vi "Hardware-RegisterControlsCalPoints.vi"(0 "User LED 1":T4, 1 "User LED 2":T4, 5 "Key [V]":sgl) -> (10 "System Settings":T5={"MPRD"=FALSE, "IO Lock MPRD Disable"=FALSE, "User LED 1"=enum."Off", "User LED 2"=enum."Off", "DI HS Fault Filter Time [s]"=1e-06, "Clamp Fault Filter Time [s]"=1e-06, "HH Shoot Through Time [s]"=1e-06, "HH ISeq Dur PS"=8, "HH Open Threshold [A]"=0.1} {"HH Open Threshold [A]" min=0 max=8 format="%#_3p"; "HH ISeq Dur PS" items=["3.3ms @ 20MHz"=0, "6.5ms @ 10MHz"=4, "13ms @ 5MHz"=6, "26ms @ 2.5MHz"=7]; "HH Shoot Through Time [s]" min=0 max=0.003277 format="%#_3p"; "Clamp Fault Filter Time [s]" min=0 max=0.003277 format="%#_3p"; "DI HS Fault Filter Time [s]" min=0 max=0.003277 format="%#_3p"}, 14 "A Configuration":T8={"Configuration"=enum."Solenoid Unipolar 4", "Power Supply Enable"=FALSE, "Boost Voltage [V]"=100.0, "Inject Enable"=FALSE, "DI Zener Enable"=FALSE, "DI Zener Voltage [V]"=0.0, "Pump Zener Enable"=FALSE, "Pump Zener Voltage [V]"=0.0, "Boost Clamp [V]"=0.0} {"Pump Zener Voltage [V]" min=0 max=240 format="%#_13g"; "DI Zener Voltage [V]" min=0 max=100 format="%#_13g"; "Boost Clamp [V]" min=0 max=220 format="%#_13g"; "Boost Voltage [V]" min=0 max=220 format="%#_13g"}, 15 "A Fault Clear":T7, 16 "B Configuration":T8={"Configuration"=enum."Solenoid Unipolar 4", "Power Supply Enable"=FALSE, "Boost Voltage [V]"=100.0, "Inject Enable"=FALSE, "DI Zener Enable"=FALSE, "DI Zener Voltage [V]"=0.0, "Pump Zener Enable"=FALSE, "Pump Zener Voltage [V]"=0.0, "Boost Clamp [V]"=0.0} {"Pump Zener Voltage [V]" min=0 max=240 format="%#_13g"; "DI Zener Voltage [V]" min=0 max=100 format="%#_13g"; "Boost Clamp [V]" min=0 max=220 format="%#_13g"; "Boost Voltage [V]" min=0 max=220 format="%#_13g"}, 17 "B Fault Clear":T7, 18 "HW|HH|Config":T3(array[cluster])=[{"Mode"=enum."Off", "IO Lock State"=FALSE, "Phase 1 FP"=FALSE, "Fault Clear"=FALSE, "ISeq"=[{"Upper [A]"=0.0, "Lower [A]"=0.0, "Duration [s]"=0.0}, {"Upper [A]"=0.0, "Lower [A]"=0.0, "Duration [s]"=0.0}]}, {"Mode"=enum."Off", "IO Lock State"=FALSE, "Phase 1 FP"=FALSE, "Fault Clear"=FALSE, "ISeq"=[{"Upper [A]"=0.0, "Lower [A]"=0.0, "Duration [s]"=0.0}, {"Upper [A]"=0.0, "Lower [A]"=0.0, "Duration [s]"=0.0}]}, {"Mode"=enum."Off", "IO Lock State"=FALSE, "Phase 1 FP"=FALSE, "Fault Clear"=FALSE, "ISeq"=[{"Upper [A]"=0.0, "Lower [A]"=0.0, "Duration [s]"=0.0}, {"Upper [A]"=0.0, "Lower [A]"=0.0, "Duration [s]"=0.0}]}, {"Mode"=enum."Off", "IO Lock State"=FALSE, "Phase 1 FP"=FALSE, "Fault Clear"=FALSE, "ISeq"=[{"Upper [A]"=0.0, "Lower [A]"=0.0, "Duration [s]"=0.0}, {"Upper [A]"=0.0, "Lower [A]"=0.0, "Duration [s]"=0.0}]}, {"Mode"=enum."Off", "IO Lock State"=FALSE, "Phase 1 FP"=FALSE, "Fault Clear"=FALSE, "ISeq"=[{"Upper [A]"=0.0, "Lower [A]"=0.0, "Duration [s]"=0.0}, {"Upper [A]"=0.0, "Lower [A]"=0.0, "Duration [s]"=0.0}]}, {"Mode"=enum."Off", "IO Lock State"=FALSE, "Phase 1 FP"=FALSE, "Fault Clear"=FALSE, "ISeq"=[{"Upper [A]"=0.0, "Lower [A]"=0.0, "Duration [s]"=0.0}, {"Upper [A]"=0.0, "Lower [A]"=0.0, "Duration [s]"=0.0}]}, {"Mode"=enum."Off", "IO Lock State"=FALSE, "Phase 1 FP"=FALSE, "Fault Clear"=FALSE, "ISeq"=[{"Upper [A]"=0.0, "Lower [A]"=0.0, "Duration [s]"=0.0}, {"Upper [A]"=0.0, "Lower [A]"=0.0, "Duration [s]"=0.0}]}, {"Mode"=enum."Off", "IO Lock State"=FALSE, "Phase 1 FP"=FALSE, "Fault Clear"=FALSE, "ISeq"=[{"Upper [A]"=0.0, "Lower [A]"=0.0, "Duration [s]"=0.0}, {"Upper [A]"=0.0, "Lower [A]"=0.0, "Duration [s]"=0.0}]}, {"Mode"=enum."Off", "IO Lock State"=FALSE, "Phase 1 FP"=FALSE, "Fault Clear"=FALSE, "ISeq"=[{"Upper [A]"=0.0, "Lower [A]"=0.0, "Duration [s]"=0.0}, {"Upper [A]"=0.0, "Lower [A]"=0.0, "Duration [s]"=0.0}]}, {"Mode"=enum."Off", "IO Lock State"=FALSE, "Phase 1 FP"=FALSE, "Fault Clear"=FALSE, "ISeq"=[{"Upper [A]"=0.0, "Lower [A]"=0.0, "Duration [s]"=0.0}, {"Upper [A]"=0.0, "Lower [A]"=0.0, "Duration [s]"=0.0}]}, {"Mode"=enum."Off", "IO Lock State"=FALSE, "Phase 1 FP"=FALSE, "Fault Clear"=FALSE, "ISeq"=[{"Upper [A]"=0.0, "Lower [A]"=0.0, "Duration [s]"=0.0}, {"Upper [A]"=0.0, "Lower [A]"=0.0, "Duration [s]"=0.0}]}, {"Mode"=enum."Off", "IO Lock State"=FALSE, "Phase 1 FP"=FALSE, "Fault Clear"=FALSE, "ISeq"=[{"Upper [A]"=0.0, "Lower [A]"=0.0, "Duration [s]"=0.0}, {"Upper [A]"=0.0, "Lower [A]"=0.0, "Duration [s]"=0.0}]}] {"ISeq"."Duration [s]" min=0 max=26 format="%#_3p"; "ISeq"."Lower [A]" min=0 max=8 format="%#_3p"; "ISeq"."Upper [A]" min=0 max=8 format="%#_3p"})   [LabVIEW 2016, in "DSI-RT.lvlib"]
uses:
  DSI-RT.lvlib
  <vilib>/Powertrain Controls/Device Drivers/DCM/Rev0/RT/Configuration.ctl
  <vilib>/Powertrain Controls/Device Drivers/DCM/Rev0/FPGA/DI - Bank Configuration.ctl
  <vilib>/Powertrain Controls/Device Drivers/DCM/Tools/FPGA/8 Channels.ctl
  <vilib>/Powertrain Controls/Device Drivers/DCM/Rev0/RT/System Settings.ctl
  <vilib>/Powertrain Controls/Device Drivers/DCM/Rev0/RT/User LED.ctl
  <vilib>/Powertrain Controls/Device Drivers/DCM/HH/RT/Duration Pre Scale.ctl
  <vilib>/Powertrain Controls/Device Drivers/DCM/HH/RT/Mode.ctl
  <vilib>/Powertrain Controls/Device Drivers/DCM/HH/RT/ISeq.ctl
  <vilib>/addons/Software Calibration Management/xSCM/CalPoint.xnode
  <vilib>/Powertrain Controls/Device Drivers/DCM/Rev0/RT/DCM - RT.lvclass
  <vilib>/Powertrain Controls/Device Drivers/DCM/HH/RT/DCM - RT - HH.lvlib
  <vilib>/addons/Software Calibration Management/xSCM/ni_scm.dll
  <vilib>/Powertrain Controls/Device Drivers/DCM/Rev0/FPGA/DCM - FPGA.lvlib
  <vilib>/Powertrain Controls/Device Drivers/DCM/Tools/FPGA/DCM - FPGA - Tools.lvlib
panel:
  # "Voltage [DV]"
  # "Voltage [V]"
  # "Voltage [DV]"
  # "Voltage [V]"
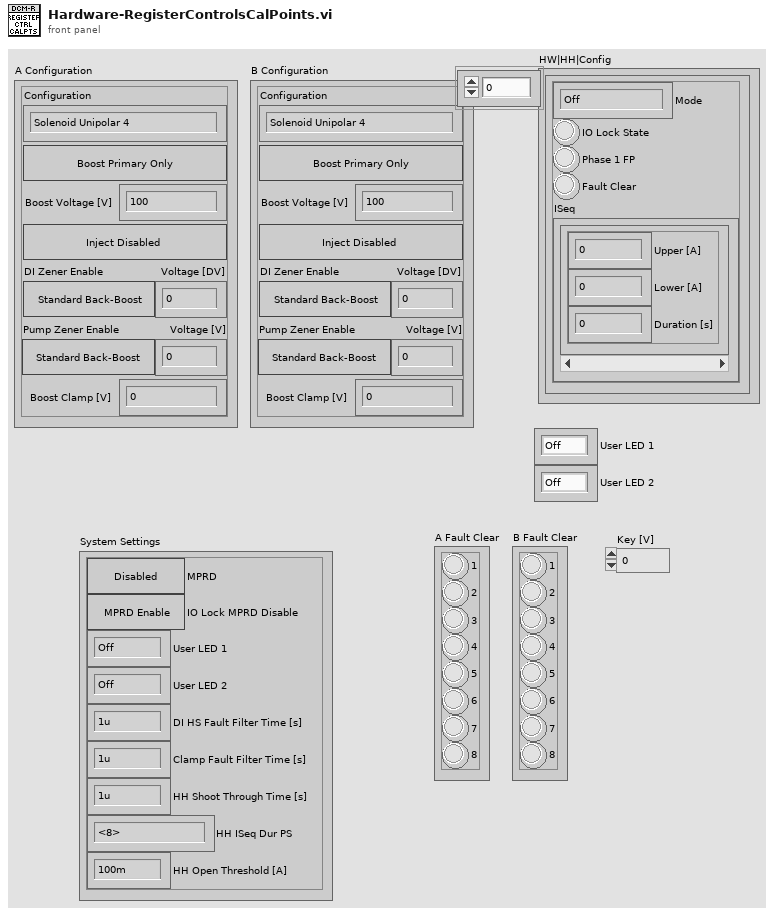
[diagram p1: front panel]
types:
  T1 = typedef "DCM - RT - HH.lvlib/Mode.ctl" = enum16{"Off", "Lowside", "Highside", "PFI", "Full H", "3-Phase"}
  T2 = typedef "DCM - RT - HH.lvlib/ISeq.ctl" = cluster{"Upper [A]":sgl, "Lower [A]":sgl, "Duration [s]":sgl}
  T3 = cluster{"Mode":T1, "IO Lock State":bool, "Phase 1 FP":bool, "Fault Clear":bool, "ISeq":T2[]}[]
  T4 = typedef "DCM - RT.lvclass/User LED.ctl" = enum16{"Off", "Yellow", "Green"}
  T5 = typedef "DCM - RT.lvclass/System Settings.ctl" = cluster{"MPRD":bool, "IO Lock MPRD Disable":bool, "User LED 1":T4, "User LED 2":T4, "DI HS Fault Filter Time [s]":sgl, "Clamp Fault Filter Time [s]":sgl, "HH Shoot Through Time [s]":sgl, "HH ISeq Dur PS":T6, "HH Open Threshold [A]":sgl}
  T6 = typedef "DCM - RT - HH.lvlib/Duration Pre Scale.ctl" = u8
  T7 = typedef "DCM - FPGA - Tools.lvlib/8 Channels.ctl" = cluster{"1":bool, "2":bool, "3":bool, "4":bool, "5":bool, "6":bool, "7":bool, "8":bool}
  T8 = typedef "DCM - RT.lvclass/Configuration.ctl" = cluster{"Configuration":T9, "Power Supply Enable":bool, "Boost Voltage [V]":sgl, "Inject Enable":bool, "DI Zener Enable":bool, "DI Zener Voltage [V]":sgl, "Pump Zener Enable":bool, "Pump Zener Voltage [V]":sgl, "Boost Clamp [V]":sgl}
  T9 = typedef "DCM - FPGA.lvlib/DI - Bank Configuration.ctl" = enum8{"Solenoid Unipolar 4", "Solenoid Unipolar 7 (Muxed)", "Solenoid Unipolar 8 (Muxed)", "Solenoid Bipolar 2", "Solenoid Bipolar 3 (Muxed)", "Piezo Unipolar 2", "Piezo Unipolar 3 (Muxed)", "Piezo Unipolar 4 (Muxed)", "Piezo Bipolar 2", "Piezo Bipolar 3 (Muxed)"}
  T10 = cluster{"Mode":enum16{"Off", "Lowside", "Highside", "PFI", "Full H", "3-Phase"}, "IO Lock State":bool, "Phase 1 FP":bool, "Fault Clear":bool, "ISeq":cluster{"Upper [A]":sgl, "Lower [A]":sgl, "Duration [s]":sgl}[]}[]
  T11 = cluster{"Boolean array[0]":bool, "Boolean array[1]":bool, "Boolean array[2]":bool, "Boolean array[3]":bool, "Boolean array[4]":bool, "Boolean array[5]":bool, "Boolean array[6]":bool, "Boolean array[7]":bool}
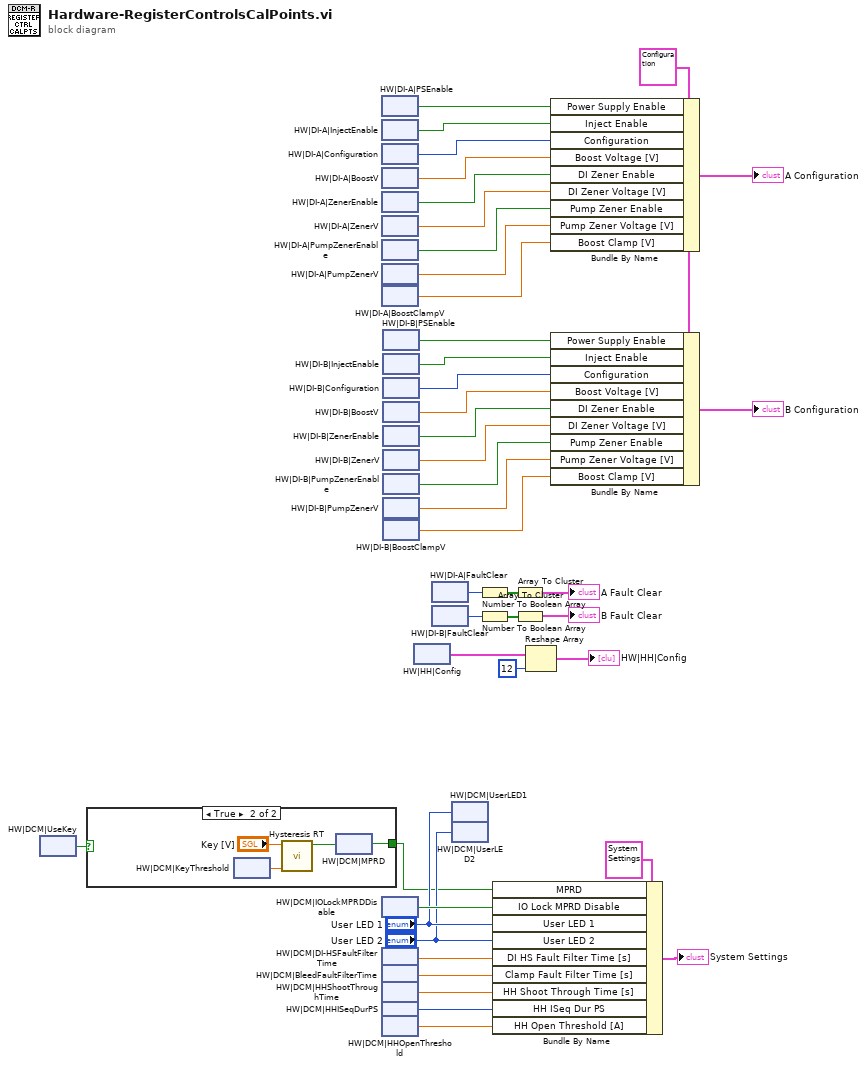
[diagram p0: block diagram]
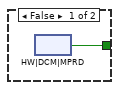
[diagram p2: hidden frame]
diagram:
  w2 = T8 {"Configuration"=enum."Solenoid Unipolar 4", "Power Supply Enable"=FALSE, "Boost Voltage [V]"=100.0, "Inject Enable"=FALSE, "DI Zener Enable"=FALSE, "DI Zener Voltage [V]"=0.0, "Pump Zener Enable"=FALSE, "Pump Zener Voltage [V]"=0.0, "Boost Clamp [V]"=0.0} ("A Configuration 2")
  n1 = xnode "HW|DCM|UseKey"() -> ("Value"=w14:bool)
  n2 = case shown="True" w14 {
    tunnel: [w43 w50] -> w1
    frame False {
      n3 = xnode "HW|DCM|MPRD"() -> ("Value"=w43:bool)
    }
    frame True {
      n4 = xnode "HW|DCM|KeyThreshold"() -> ("Value"=w49:sgl)
      n5 = call "Hysteresis RT.vi"("Threshold [V] (7)"=w49, "Switch [V]"="Key [V]") -> ("State"=w50:bool)  [unwired: 9 in]
      n6 = xnode "HW|DCM|MPRD"("Value"=w50) -> ()
    }
  }
  n7 = xnode "HW|DI-A|PSEnable"() -> ("Value"=w12:bool)
  n8 = xnode "HW|DI-A|InjectEnable"() -> ("Value"=w11:bool)
  n9 = xnode "HW|DI-A|Configuration"() -> ("Value"=w10:u8)
  n10 = xnode "HW|DI-A|BoostV"() -> ("Value"=w9:sgl)
  n11 = xnode "HW|DI-A|ZenerEnable"() -> ("Value"=w8:bool)
  n12 = xnode "HW|DI-A|ZenerV"() -> ("Value"=w7:sgl)
  n13 = xnode "HW|DI-A|PumpZenerEnable"() -> ("Value"=w6:bool)
  n14 = xnode "HW|DI-A|PumpZenerV"() -> ("Value"=w5:sgl)
  n15 = xnode "HW|DI-A|BoostClampV"() -> ("Value"=w4:sgl)
  n16 = xnode "HW|DCM|IOLockMPRDDisable"() -> ("Value"=w26:bool)
  n17 = xnode "HW|DCM|DI-HSFaultFilterTime"() -> ("Value"=w33:sgl)
  n18 = xnode "HW|DCM|BleedFaultFilterTime"() -> ("Value"=w31:sgl)
  n19 = xnode "HW|DCM|HHShootThroughTime"() -> ("Value"=w32:sgl)
  n20 = xnode "HW|DCM|HHISeqDurPS"() -> ("Value"=w30:u8)
  n21 = xnode "HW|DCM|HHOpenThreshold"() -> ("Value"=w29:sgl)
  n22 = xnode "HW|DI-B|PSEnable"() -> ("Value"=w38:bool)
  n23 = xnode "HW|DI-B|InjectEnable"() -> ("Value"=w37:bool)
  n24 = xnode "HW|DI-B|Configuration"() -> ("Value"=w18:u8)
  n25 = xnode "HW|DI-B|BoostV"() -> ("Value"=w36:sgl)
  n26 = xnode "HW|DI-B|ZenerEnable"() -> ("Value"=w35:bool)
  n27 = xnode "HW|DI-B|ZenerV"() -> ("Value"=w34:sgl)
  n28 = xnode "HW|DI-B|PumpZenerEnable"() -> ("Value"=w13:bool)
  n29 = xnode "HW|DI-B|PumpZenerV"() -> ("Value"=w28:sgl)
  n30 = xnode "HW|DI-B|BoostClampV"() -> ("Value"=w27:sgl)
  n31 = xnode "HW|HH|Config"() -> ("Value"=w15:T10)
  n32 = xnode "HW|DI-A|FaultClear"() -> ("Value"=w41:u8)
  n33 = xnode "HW|DI-B|FaultClear"() -> ("Value"=w42:u8)
  n34 = xnode "HW|DCM|UserLED1"("Value"="User LED 1") -> ()
  n35 = xnode "HW|DCM|UserLED2"("Value"="User LED 2") -> ()
  n36 = Number To Boolean Array(number=w41) -> (Boolean array=w40:bool[])
  n37 = Number To Boolean Array(number=w42) -> (Boolean array=w39:bool[])
  n38 = Bundle By Name(cluster=T5 {"MPRD"=FALSE, "IO Lock MPRD Disable"=FALSE, "User LED 1"=enum."Off", "User LED 2"=enum."Off", "DI HS Fault Filter Time [s]"=1e-06, "Clamp Fault Filter Time [s]"=1e-06, "HH Shoot Through Time [s]"=1e-06, "HH ISeq Dur PS"=8, "HH Open Threshold [A]"=0.1} ("System Settings 2"), "MPRD"=w1, "IO Lock MPRD Disable"=w26, "User LED 1"="User LED 1", "User LED 2"="User LED 2", "DI HS Fault Filter Time [s]"=w33, "Clamp Fault Filter Time [s]"=w31, "HH Shoot Through Time [s]"=w32, "HH ISeq Dur PS"=w30, "HH Open Threshold [A]"=w29) -> (→"System Settings":T5)
  n39 = Array To Cluster(array=w40) -> (cluster=→"A Fault Clear":T11)
  n40 = Array To Cluster(array=w39) -> (cluster=→"B Fault Clear":T11)
  n41 = Reshape Array(w15, 12 ("dimension size")) -> (→"HW|HH|Config":T10)
  n42 = Bundle By Name(cluster=w2, "Power Supply Enable"=w12, "Inject Enable"=w11, "Configuration"=w10, "Boost Voltage [V]"=w9, "DI Zener Enable"=w8, "DI Zener Voltage [V]"=w7, "Pump Zener Enable"=w6, "Pump Zener Voltage [V]"=w5, "Boost Clamp [V]"=w4) -> (→"A Configuration":T8)
  n43 = Bundle By Name(cluster=w2, "Power Supply Enable"=w38, "Inject Enable"=w37, "Configuration"=w18, "Boost Voltage [V]"=w36, "DI Zener Enable"=w35, "DI Zener Voltage [V]"=w34, "Pump Zener Enable"=w13, "Pump Zener Voltage [V]"=w28, "Boost Clamp [V]"=w27) -> (→"B Configuration":T8)
